vi "Attributes.vi"(11 "Type in":refnum<class "Type.lvclass">) -> (2 "Attributes":T1)   [LabVIEW 2020, in "Conditu2.lvlib" / "Columns.lvlib" / "Type.lvclass"]
uses:
  Type.lvclass
  Attributes.ctl
  Type.lvclass/Type.ctl
  Conditu2.lvlib
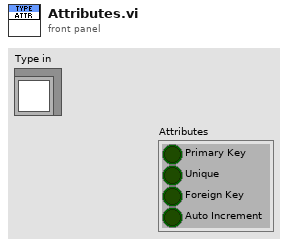
[diagram p1: front panel]
types:
  T1 = typedef "Conditu2.lvlib/Attributes.ctl" = cluster{"Primary Key":bool, "Unique":bool, "Foreign Key":bool, "Auto Increment":bool}
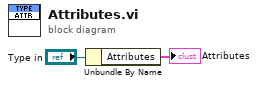
[diagram p0: block diagram]
diagram:
  n1 = Unbundle By Name("Type in") -> ("Attributes"=→"Attributes":T1)
